vi "Car_Speed_R128F.vi"(10 "精度":dbl=0.0625, 11 "车速":u16) -> (3 "报文":T1 {"[7]" format="%02x"; "[6]" format="%02x"; "[5]" format="%02x"; "[4]" format="%02x"; "[3]" format="%02x"; "[2]" format="%02x"; "[1]" format="%02x"; "[0]" format="%02x"})   [LabVIEW 2020]
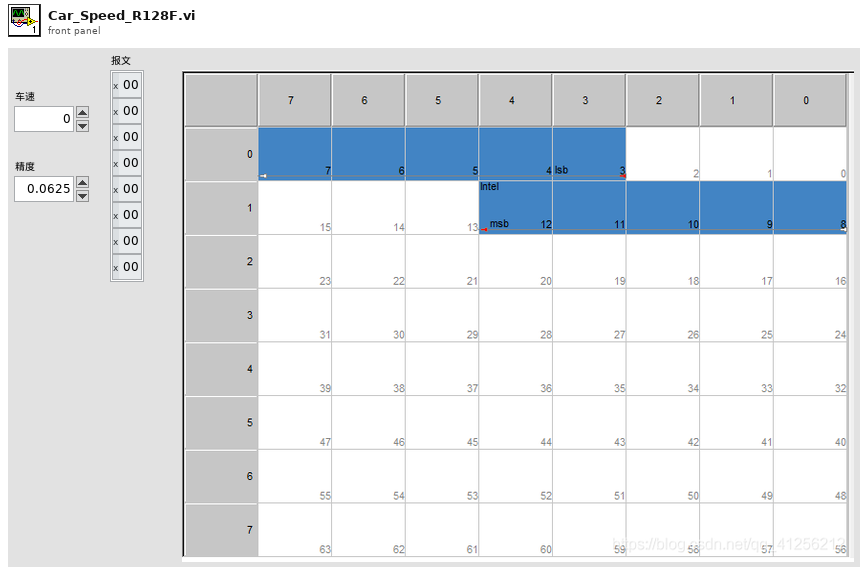
[diagram p1: front panel]
types:
  T1 = cluster{"[0]":u8, "[1]":u8, "[2]":u8, "[3]":u8, "[4]":u8, "[5]":u8, "[6]":u8, "[7]":u8}
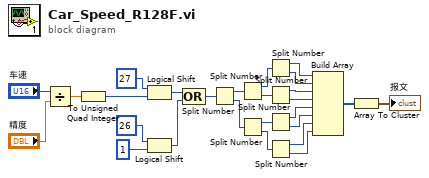
[diagram p0: block diagram]
diagram:
  n1 = Divide(x="车速", y="精度") -> (x/y=w23:dbl)
  n2 = To Unsigned Quad Integer(1:w23) -> (0:w5:u64)
  n3 = Logical Shift(y=i16 27, x=w5) -> (x << y=w13:u64)
  n4 = Logical Shift(y=i16 26, x=u64 1) -> (x << y=w15:u64)
  n5 = Compound Arithmetic op=OR ("复合运算")(w13, w15) -> (w12:u64)
  n6 = Split Number(x=w12) -> (hi(x)=w21:u32, lo(x)=w20:u32)
  n7 = Split Number(x=w21) -> (hi(x)=w19:u16, lo(x)=w18:u16)
  n8 = Split Number(x=w20) -> (hi(x)=w17:u16, lo(x)=w3:u16)
  n9 = Split Number(x=w19) -> (hi(x)=w11:u8, lo(x)=w10:u8)
  n10 = Split Number(x=w18) -> (hi(x)=w9:u8, lo(x)=w8:u8)
  n11 = Split Number(x=w17) -> (hi(x)=w7:u8, lo(x)=w6:u8)
  n12 = Split Number(x=w3) -> (hi(x)=w2:u8, lo(x)=w1:u8)
  n13 = Build Array(w11, w10, w9, w8, w7, w6, w2, w1) -> (w4:u8[])
  n14 = Array To Cluster(array=w4) -> (cluster=→"报文":T1)
